vi "Setup Auto.vi"() -> (3 "Auto Data":T1)   [LabVIEW 2025]
uses:
  Drive/Implementation/Auto Data.ctl
  swerve-template/Type Definitions/Data/Robot Velocities.ctl
  Drive Conditions.ctl
  239c1ceb-589e-4f7c-8125-dfea88b83b5c.vi
  <vilib>/Rock Robotics/Network Tables/NT Read String.vi
  <vilib>/Rock Robotics/Network Tables/NT Read String Array.vi
  <vilib>/Utility/file.llb/Read Delimited Spreadsheet (string).vi
  Robot Global Data.vi
  <vilib>/Rock Robotics/Network Tables/NT Read Boolean.vi
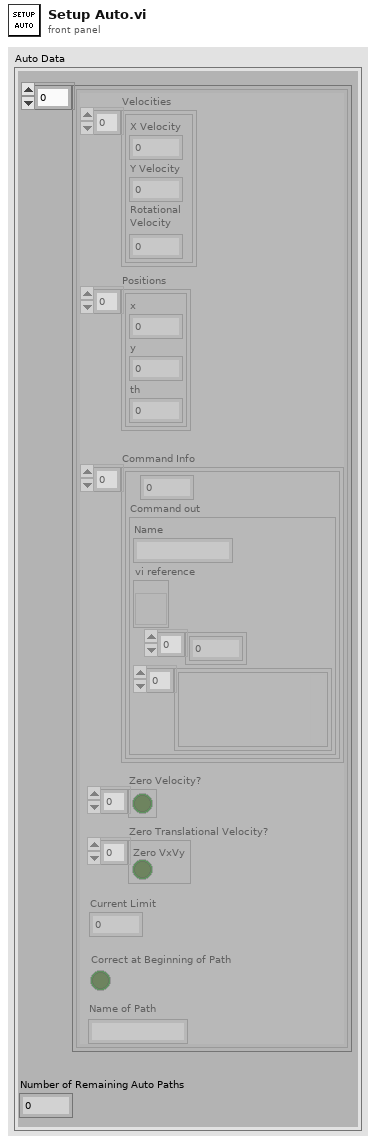
[diagram p1: front panel]
types:
  T1 = typedef "Auto Data.ctl" = cluster{"Auto Data":cluster{"Velocities":T2[], "Positions":cluster{"x":dbl, "y":dbl, "th":dbl}[], "Command Info":cluster{dbl, "Command out":cluster{"Name":string, "vi reference":refnum<vi>, i32[], variant[]}}[], "Zero Velocity?":bool[], "Zero Translational Velocity?":bool[], "Current Limit":dbl, "Correct at Beginning of Path":bool, "Name of Path":string}[], "Number of Remaining Auto Paths":dbl}
  T2 = typedef "Robot Velocities.ctl" = cluster{"X Velocity":dbl, "Y Velocity":dbl, "Rotational \nVelocity":dbl}
  T3 = typedef "Drive Conditions.ctl" = cluster{"Field Centric":bool, "BotPose Correction":bool, "Theta Align":cluster{"Theta Align":bool, "Type":enum16{"Hub", "Corner of Field"}}, "Reset PIDs":bool, "Align to Field":cluster{"Align to Bump or Shoot":bool, "Field Element":enum16{"Bump", "Shooter Shot", "Trench"}}}
  T4 = typedef "Single Cmd Info.ctl" = cluster{"Name":string, "CPTM.DataType":variant, "All Control Values Variant":cluster{"Name":string, "Variant Data":variant}[], "icon full":T5, "icon scaled":T5, "Path":path, "Subsystem Color":u32}
  T5 = typedef "imagedata.ctl" = cluster{"image type":i32, "image depth":i32, "image":u8[], "mask":u8[], "colors":u32[], "Rectangle":cluster{"left":i16, "top":i16, "right":i16, "bottom":i16}}
  T6 = cluster{"Name":string, "vi reference":refnum<vi>, i32[], variant[]}
  T7 = cluster{"Time (s)":dbl, "Command out":cluster{"Name":string, "vi reference":refnum<vi>, i32[], variant[]}}
  T8 = cluster{"Time (s)":dbl, "Command out":cluster{"Name":string, "vi reference":refnum<vi>, i32[], variant[]}}[]
  T9 = cluster{"Velocities":T2[], "Positions":cluster{"x":dbl, "y":dbl, "th":dbl}[], cluster{"Time (s)":dbl, "Command out":cluster{"Name":string, "vi reference":refnum<vi>, i32[], variant[]}}[], "Zero Velocity?":bool[], "Zero Translational Velocity?":bool[], "Current Limit":dbl, "Correct at Beginning \nof Path":bool, "String":string}
  T10 = cluster{cluster{"Velocities":T2[], "Positions":cluster{"x":dbl, "y":dbl, "th":dbl}[], cluster{"Time (s)":dbl, "Command out":cluster{"Name":string, "vi reference":refnum<vi>, i32[], variant[]}}[], "Zero Velocity?":bool[], "Zero Translational Velocity?":bool[], "Current Limit":dbl, "Correct at Beginning \nof Path":bool, "String":string}[], i32}
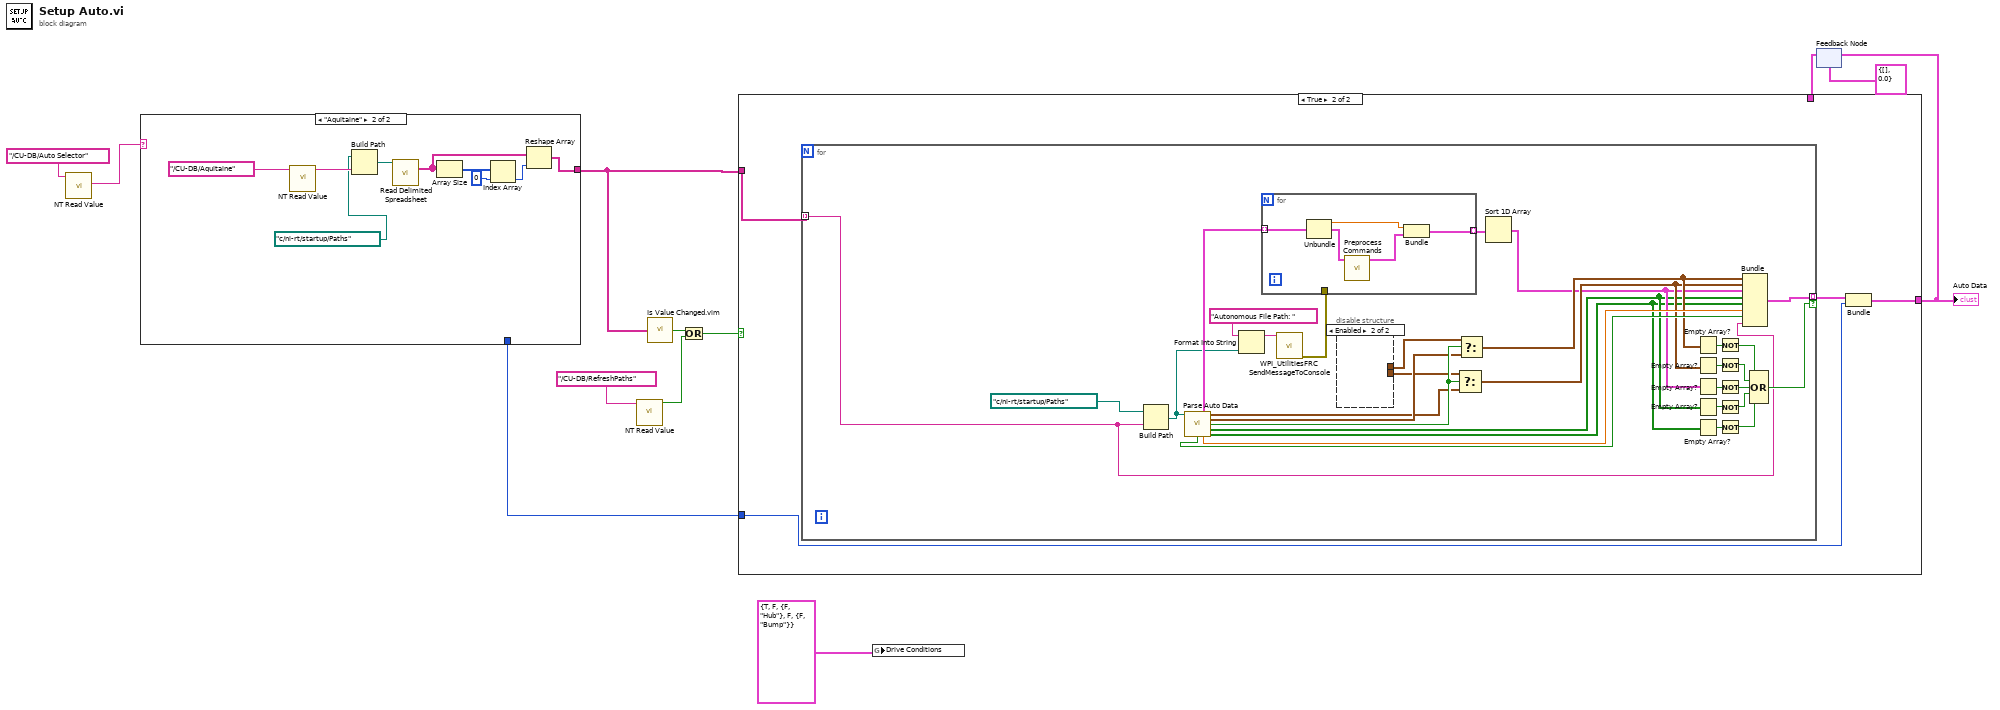
[diagram p0: block diagram]
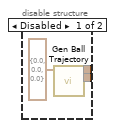
[diagram p3: hidden frame]
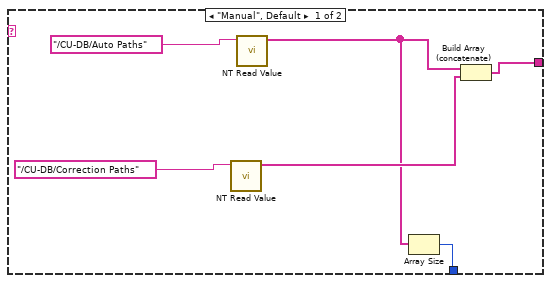
[diagram p4: hidden frame]
diagram:
  n1 = call-poly <vilib>:"NT Read Value.vi"("name"="/CU-DB/Auto Selector") -> ("value"=w12:string)  [unwired: 8 in, 2 out]
  n2 = case shown="\"Aquitaine\"" w12 {
    tunnel: [w15 w20] -> w9
    tunnel: [w13 _] -> w3
    frame "Manual", Default {
      n3 = call-poly <vilib>:"NT Read Value.vi"("name"="/CU-DB/Correction Paths") -> ("value"=w16:string[])  [unwired: 8 in, 2 out]
      n4 = call-poly <vilib>:"NT Read Value.vi"("name"="/CU-DB/Auto Paths") -> ("value"=w14:string[])  [unwired: 8 in, 2 out]
      n5 = Array Size(array=w14) -> (size(s)=w13:i32)
      n6 = Build Array (concatenate)(w14, w16) -> (w15:string[])
    }
    frame "Aquitaine" {
      n7 = call-poly <vilib>:"NT Read Value.vi"("name"="/CU-DB/Aquitaine") -> ("value"=w26:string)  [unwired: 8 in, 2 out]
      n8 = Build Path(base path=path "c:/ni-rt/startup/Paths" ("appended path"), name or relative path=w26) -> (appended path=w25:path)
      n9 = call-poly <vilib>:"Read Delimited Spreadsheet.vi"("file path (dialog if empty)"=w25) -> ("all rows"=w21:string[][])  [unwired: 9 in, 5 out]
      n10 = Array Size(array=w21) -> (size(s)=w24:i32[])
      n11 = Index Array(array=w24, index=0) -> (element=w22:i32)
      n12 = Reshape Array(w21, w22) -> (w20:string[])
    }
  }
  n13 = call-poly <vilib>:"NT Read Value.vi"("name"="/CU-DB/RefreshPaths" ("Name")) -> ("value"=w5:bool)  [unwired: 8 in, 2 out]
  n14 = call "Is Value Changed.vim"("value"=w9) -> ("changed or first call?"=w6:bool)
  n15 = Or(x=w6, y=w5) -> (x .or. y?=w4:bool)
  n16 = global write "Robot Global Data.vi" "Drive Conditions"(T3 {"Field Centric"=TRUE, "BotPose Correction"=FALSE, "Theta Align"={"Theta Align"=FALSE, "Type"=enum."Hub"}, "Reset PIDs"=FALSE, "Align to Field"={"Align to Bump or Shoot"=FALSE, "Field Element"=enum."Bump"}} ("Drive Conditions")) -> ()
  n17 = feedback #1(T1 {"Auto Data"=[], "Number of Remaining Auto Paths"=0.0} ("Cluster")) -> (w8:T1)
  n18 = case shown="True" w4 {
    tunnel: [w28 w29] -> w1
    tunnel: w9 -> [_ w32]
    tunnel: w8 -> [w28 _]
    tunnel: w3 -> [_ w30]
    frame False {
    }
    frame True {
      n19 = for {
        tunnel: w32 -> [w33] mode=indexing
        tunnel: [w50] -> w31 mode=indexing if=w34
        n20 = Build Path(base path=path "c:/ni-rt/startup/Paths" ("appended path"), name or relative path=w33) -> (appended path=w63:path)
        n21 = call "Parse Auto Data.vi"("path"=w63) -> ("Commands out"=w64:cluster{"Time (s)":dbl, T4, bool}[], "Positions"=w56:cluster{"x":dbl, "y":dbl, "th":dbl}[], "Velocities"=w58:T2[], "Ball Pickup"=w60:bool, "Zero Velocity?"=w46:bool[], "Correct at Beginning \nof Path"=w51:bool, "Current Limit"=w52:dbl, "Zero Translational Velocity?"=w45:bool[])  [unwired: 6 in, 1 out]
        n22 = Format Into String(initial string="Autonomous File Path: ", w63) -> (resulting string=w62:string)  [unwired: 2 in, 1 out]
        n23 = call <vilib>:"WPI_UtilitiesFRC SendMessageToConsole.vi"("Message"=w62) -> ("error out"=w55:errorcluster)  [unwired: 14 in]
        n24 = for {
          tunnel: w64 -> [w71] mode=indexing
          tunnel: [w68] -> w54 mode=indexing
          tunnel: w55 -> [_]
          n25 = Unbundle(w71) -> ("Time (s)"=w72:dbl, w70:T4)  [unwired: 1 out]
          n26 = call "Preprocess Commands.vi"("Command In"=w70) -> ("Command out"=w69:T6)  [unwired: 10 in]
          n27 = Bundle("Time (s)"=w72, "Command out"=w69) -> (w68:T7)  [unwired: 1 in]
        }
        n28 = disable-structure shown="Enabled" {
          disable-tunnel: [w66 _] -> w59
          disable-tunnel: [w65 _] -> w57
          frame Disabled {
            n29 = call "Gen Ball Trajectory.vi"("Robot Velocities"=T2 {"X Velocity"=0.0, "Y Velocity"=0.0, "Rotational \nVelocity"=0.0}) -> ("Auto Positions"=w65:cluster{"x":dbl, "y":dbl, dbl}[], "Auto Velocities"=w66:cluster{"x out":dbl, "y out":dbl, "Omega":dbl}[])  [unwired: 9 in]
          }
          frame Enabled {
          }
        }
        n30 = Select(t=w57, s=w60, f=w56) -> (s? t:f=w48:cluster{"x":dbl, "y":dbl, "th":dbl}[])
        n31 = Select(t=w59, s=w60, f=w58) -> (s? t:f=w49:T2[])
        n32 = Sort 1D Array(array=w54) -> (sorted array=w47:T8)
        n33 = Empty Array?(array=w49) -> (empty?=w44:bool)
        n34 = Empty Array?(array=w48) -> (empty?=w43:bool)
        n35 = Empty Array?(array=w47) -> (empty?=w42:bool)
        n36 = Empty Array?(array=w46) -> (empty?=w41:bool)
        n37 = Empty Array?(array=w45) -> (empty?=w40:bool)
        n38 = Not(x=w44) -> (.not. x?=w37:bool)
        n39 = Not(x=w43) -> (.not. x?=w38:bool)
        n40 = Not(x=w42) -> (.not. x?=w39:bool)
        n41 = Not(x=w41) -> (.not. x?=w36:bool)
        n42 = Not(x=w40) -> (.not. x?=w35:bool)
        n43 = Bundle("Velocities"=w49, "Positions"=w48, w47, "Zero Velocity?"=w46, "Zero Translational Velocity?"=w45, "Current Limit"=w52, "Correct at Beginning \nof Path"=w51, "String"=w33) -> (w50:T9)  [unwired: 1 in]
        n44 = Compound Arithmetic op=OR(w37, w38, w39, w36, w35) -> (w34:bool)
      }
      n45 = Bundle(w31, w30) -> (w29:T10)  [unwired: 1 in]
    }
  }
  "Auto Data" <- w1
  n46 = feedback-in #1(w1) -> ()
